vi "TackingSailSuggestion.vi"(8 "RobotHeading":dbl, 9 "DesiredHeading":dbl, 10 "ApparentWindAngle":dbl, 11 "AbsoluteWindAngle":dbl) -> (3 "Suggested Sail Setpoints":T1 {"MainSailSuggestion" min=0.0 max=1.0; "JibSailSuggestion" min=0.0 max=1.0})   [LabVIEW 2013]
doc: "This VI should output sail and rudder instructions for how to tack across the wind. Inputs could include wind direction, robot heading, desired heading, and others of interest. Algorithm currently undetermined, ask sailors for tack thought process and communicate with the forebrain programmers to figure out when the boat will be considered in a tack and when it will be considered out of one. See JibeSailSuggestion.vi for comparison.\nEric Schneider and Bonnie Ishiguro, Jan. 2014\nThis VI has a series of steps for a tack based on the position relative to the wind. It may choose to maintain the main and jib position, or coerce them into a range. Rudder suggestion as yet undetermined, could use the PID controller to the waypoint.\nMichael Bocamazo, 2014/02/01"
uses:
  Data/TypeDefs/Sail Set Suggestions.ctl
  Utilities/Math/Angles/Angle/Angle.lvclass
panel:
  in  "Current Main Position":dbl
  in  "Current Jib Position":dbl
  in  "WindSpeed":dbl
  # "THIS IS UNUSED AT THE MOMENT"
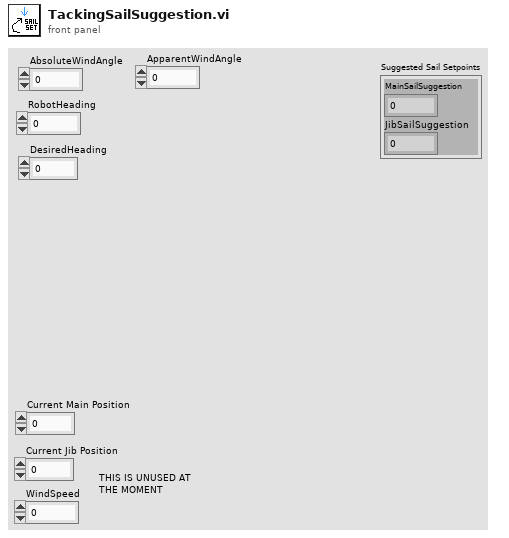
[diagram p1: front panel]
types:
  T1 = typedef "Sail Set Suggestions.ctl" = cluster{"MainSailSuggestion":dbl, "JibSailSuggestion":dbl}
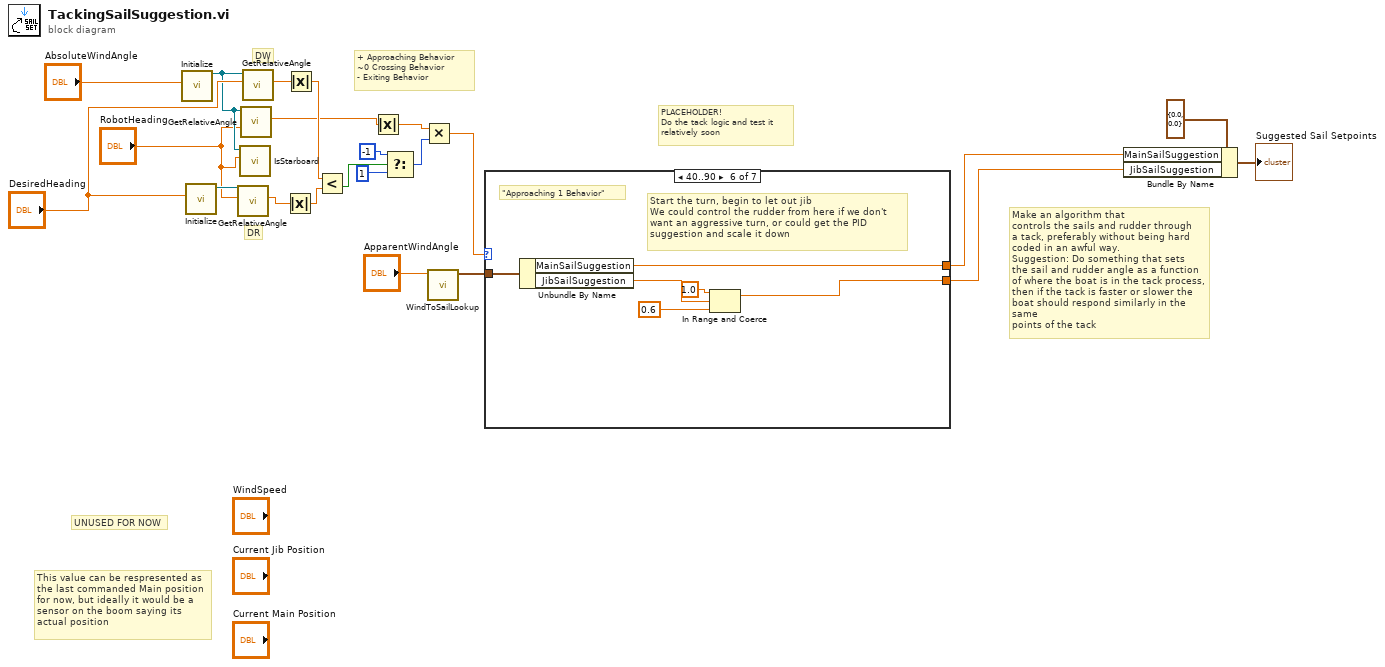
[diagram p0: block diagram]
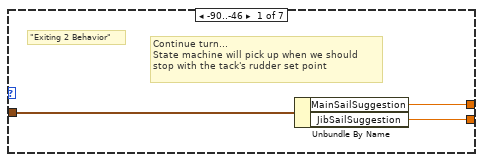
[diagram p2: hidden frame]
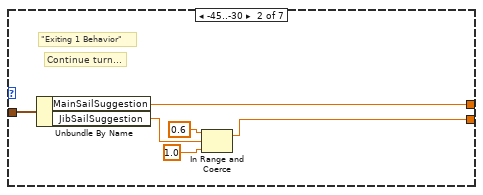
[diagram p3: hidden frame]
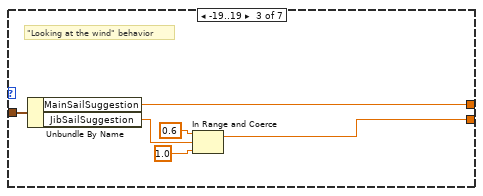
[diagram p4: hidden frame]
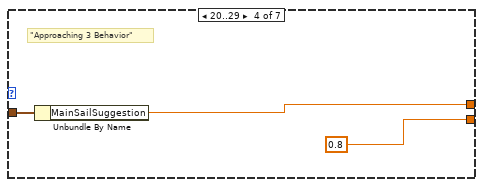
[diagram p5: hidden frame]
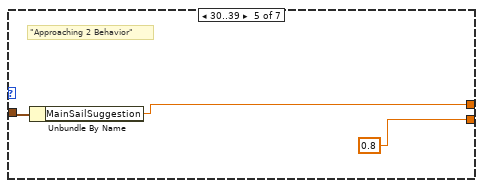
[diagram p6: hidden frame]
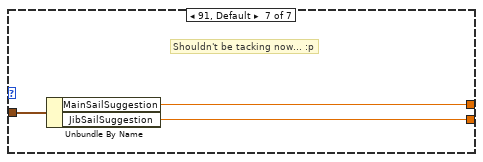
[diagram p7: hidden frame]
diagram:
  # "UNUSED FOR NOW"
  # "This value can be respresented as the last commanded Main position for now, but ideally it would be a sensor on the boom saying its actual position"
  # "Make an algorithm that\ncontrols the sails and rudder through\na tack, preferably without being hard\ncoded in an awful way.\nSuggestion: Do something that sets\nthe sail and rudder angle as a function\nof where the boat is in the tack process,\nthen if the tack is faster or slower the\nboat should respond similarly in the same\npoints of the tack"
  # "DW"
  # "DR"
  # "+ Approaching Behavior\n~0 Crossing Behavior\n- Exiting Behavior"
  # "PLACEHOLDER!\nDo the tack logic and test it\nrelatively soon"
  n1 = call "Initialize.vi"("Input Angle (Deg.)"="AbsoluteWindAngle") -> ("Angle out"=w4:refnum<class "Angle.lvclass">)  [unwired: 9 in, 1 out]
  n2 = call "Initialize.vi"("Input Angle (Deg.)"="DesiredHeading") -> ("Angle out"=w19:refnum<class "Angle.lvclass">)  [unwired: 9 in, 1 out]
  n3 = call "GetRelativeAngle.vi"("Boat Heading (Deg.)"="RobotHeading", "Angle in"=w19) -> ("Relative Angle FROM P2 TO P1 (deg)"=w8:dbl)  [unwired: 6 in, 3 out]
  n4 = call "IsStarboard.vi"("Boat Heading (Deg.)"="RobotHeading", "Angle in"=w4) -> ()  [unwired: 8 in, 2 out]
  n5 = call "GetRelativeAngle.vi"("Boat Heading (Deg.)"="RobotHeading", "Angle in"=w4) -> ("Relative Angle FROM P2 TO P1 (deg)"=w6:dbl)  [unwired: 6 in, 3 out]
  n6 = call "GetRelativeAngle.vi"("Boat Heading (Deg.)"="DesiredHeading", "Angle in"=w4) -> ("Relative Angle FROM P2 TO P1 (deg)"=w10:dbl)  [unwired: 6 in, 3 out]
  n7 = Absolute Value(x=w8) -> (abs(x)=w7:dbl)
  n8 = Absolute Value(x=w10) -> (abs(x)=w9:dbl)
  n9 = Less?(x=w9, y=w7) -> (x < y?=w11:bool)
  n10 = Absolute Value(x=w6) -> (abs(x)=w5:dbl)
  n11 = Select(t=-1, s=w11, f=1) -> (s? t:f=w14:i32)
  n12 = Multiply(x=w5, y=w14) -> (x*y=w12:dbl)
  n13 = call "WindToSailLookup.vi"("ApparentWindAngle"="ApparentWindAngle") -> ("Suggested Sail Setpoints"=w1:T1)  [unwired: 10 in]
  n14 = case shown="40..90" w12 {
    tunnel: [w24 w26 w32 w38 w41 w44 w51] -> w16
    tunnel: [w23 w27 w33 0.8 0.8 w45 w50] -> w15
    tunnel: w1 -> [w25 w28 w37 w39 w42 w47 w52]
    frame -90..-46 {
      # "Continue turn...\nState machine will pick up when we should stop with the tack's rudder set point"
      # "\"Exiting 2 Behavior\""
      n15 = Unbundle By Name(w25) -> ("MainSailSuggestion"=w24:dbl, "JibSailSuggestion"=w23:dbl)
    }
    frame -45..-30 {
      # "Continue turn..."
      # "\"Exiting 1 Behavior\""
      n16 = Unbundle By Name(w28) -> ("MainSailSuggestion"=w26:dbl, "JibSailSuggestion"=w29:dbl)
      n17 = In Range and Coerce(upper limit=0.6, x=w29, lower limit=1.0) -> (coerced(x)=w27:dbl)  [unwired: 1 out]
    }
    frame -19..19 {
      # "\"Looking at the wind\" behavior"
      n18 = Unbundle By Name(w37) -> ("MainSailSuggestion"=w32:dbl, "JibSailSuggestion"=w34:dbl)
      n19 = In Range and Coerce(upper limit=0.6, x=w34, lower limit=1.0) -> (coerced(x)=w33:dbl)  [unwired: 1 out]
    }
    frame 20..29 {
      # "\"Approaching 3 Behavior\""
      n20 = Unbundle By Name(w39) -> ("MainSailSuggestion"=w38:dbl)
    }
    frame 30..39 {
      # "\"Approaching 2 Behavior\""
      n21 = Unbundle By Name(w42) -> ("MainSailSuggestion"=w41:dbl)
    }
    frame 40..90 {
      # "Start the turn, begin to let out jib\nWe could control the rudder from here if we don't want an aggressive turn, or could get the PID suggestion and scale it down"
      # "\"Approaching 1 Behavior\""
      n22 = Unbundle By Name(w47) -> ("MainSailSuggestion"=w44:dbl, "JibSailSuggestion"=w46:dbl)
      n23 = In Range and Coerce(upper limit=1.0, x=w46, lower limit=0.6) -> (coerced(x)=w45:dbl)  [unwired: 1 out]
    }
    frame 91, Default {
      # "Shouldn't be tacking now... :p"
      n24 = Unbundle By Name(w52) -> ("MainSailSuggestion"=w51:dbl, "JibSailSuggestion"=w50:dbl)
    }
  }
  n25 = Bundle By Name(cluster=T1 {"MainSailSuggestion"=0.0, "JibSailSuggestion"=0.0} ("output cluster"), "MainSailSuggestion"=w16, "JibSailSuggestion"=w15) -> (→"Suggested Sail Setpoints":T1)
